vi "FoundValueByKey.vi"(8 "error in (no error)":errorcluster, 10 "key":string="folder", 11 "keyValues":cluster{"key":string, "value":string}[](array[cluster])) -> (0 "error out":errorcluster, 1 "found?":bool, 2 "value":string, 3 "keyValues (dup)":cluster{"key":string, "value":string}[](array[cluster]))   [LabVIEW 2014, in "OPCUA XML.lvlib"]
uses:
  OPCUA XML.lvlib
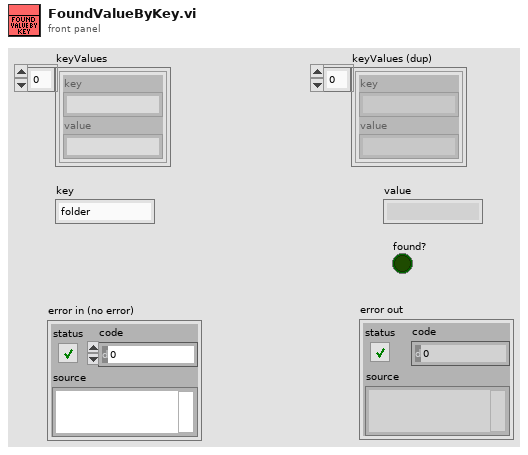
[diagram p1: front panel]
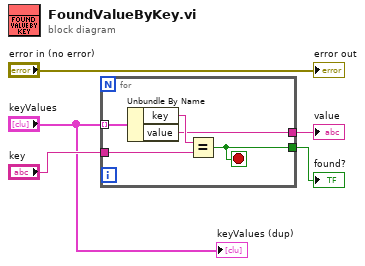
[diagram p0: block diagram]
diagram:
  n1 = for {
    tunnel: "keyValues" -> [w10] mode=indexing
    tunnel: "key" -> [w8]
    tunnel: [w7] -> w3
    tunnel: [w6] -> w4
    stop <- w6 stop-if-true
    n2 = Unbundle By Name(w10) -> ("key"=w9:string, "value"=w7:string)
    n3 = Equal?(x=w9, y=w8) -> (x = y?=w6:bool)
  }
  "found?" <- w4
  "value" <- w3
  "error out" <- "error in (no error)"
  "keyValues (dup)" <- "keyValues"
